vi "Compensazione.vi"(0 "Grandezza target":dbl, 1 "Grandezza reale letta":dbl, 2 "Precisione":dbl, 3 "Delta compensazione max":dbl, 4 "Time attesa stabilizzazione (s)":dbl, 5 "Grandezza attuale in":dbl, 6 "Reset comp?":bool, 7 "Compensazione abilitata":bool) -> (15 "compensazione":dbl, 17 "Grandezza stabilizz?":bool, 19 "Grandezza attuale out":dbl)   [LabVIEW 2019]
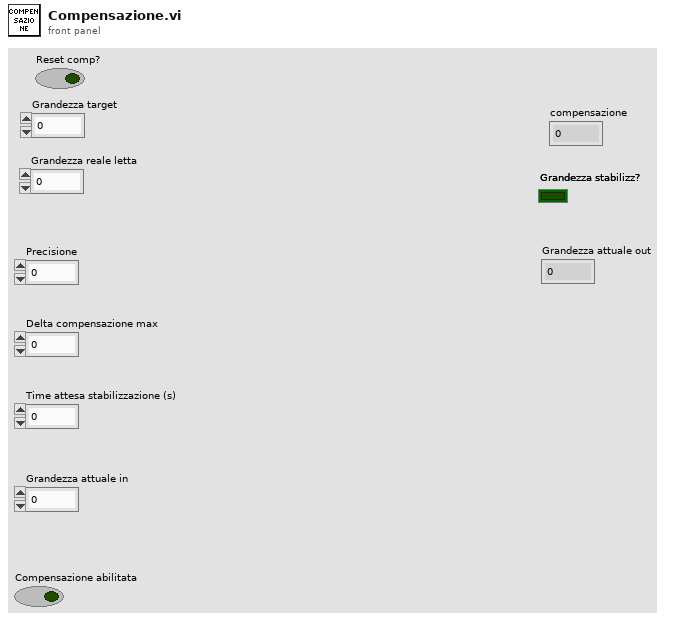
[diagram p1: front panel]
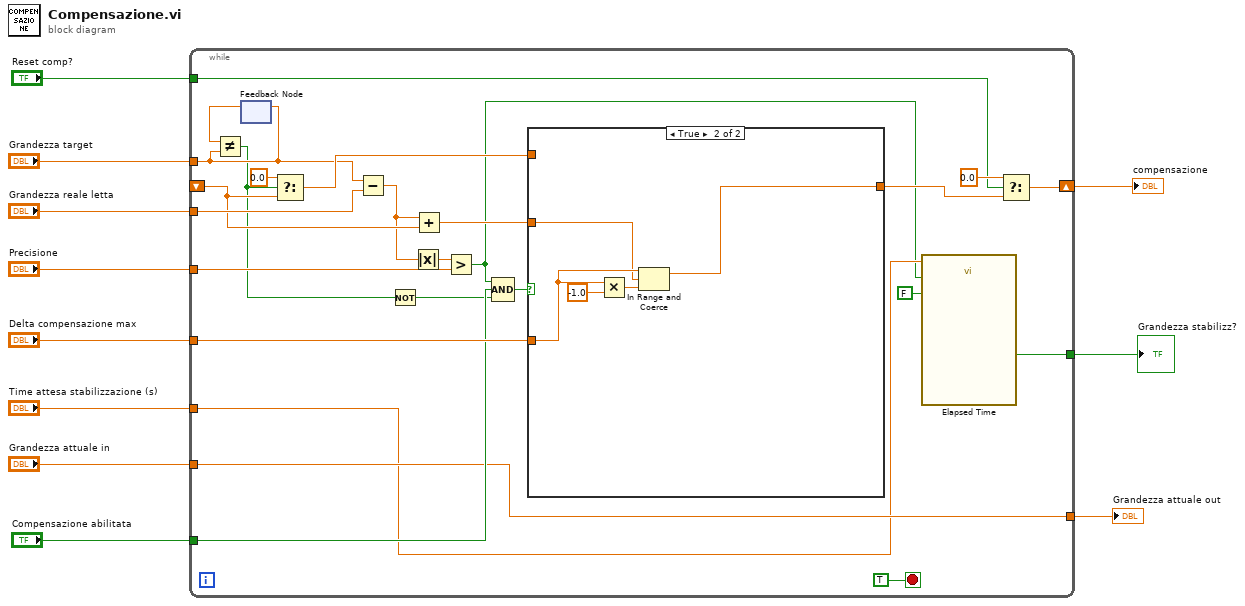
[diagram p0: block diagram]
diagram:
  n1 = while {
    tunnel: "Precisione" -> [w36]
    tunnel: "Grandezza attuale in" -> [w30]
    tunnel: "Compensazione abilitata" -> [w32]
    shift-right: [w21] -> w7
    shift-left: _ -> [w17]
    tunnel: "Delta compensazione max" -> [w34]
    tunnel: [w30] -> w6
    tunnel: "Grandezza target" -> [w18]
    tunnel: "Grandezza reale letta" -> [w29]
    tunnel: "Time attesa stabilizzazione (s)" -> [w27]
    tunnel: [w26] -> w2
    tunnel: "Reset comp?" -> [w19]
    stop <- TRUE stop-if-true
    n2 = feedback-in #1(w18) -> ()
    n3 = feedback #1() -> (w25:dbl)  [unwired: 1 in]
    n4 = Not Equal?(x=w25, y=w18) -> (x != y?=w14:bool)
    n5 = Select(t=0.0, s=w14, f=w17) -> (s? t:f=w24:dbl)
    n6 = Subtract(x=w18, y=w29) -> (x-y=w16:dbl)
    n7 = Not(x=w14) -> (.not. x?=w13:bool)
    n8 = Absolute Value(x=w16) -> (abs(x)=w33:dbl)
    n9 = Add(x=w16, y=w17) -> (x+y=w15:dbl)
    n10 = Greater?(x=w33, y=w36) -> (0:w12:bool)
    n11 = Compound Arithmetic op=AND(w12, w32, w13) -> (w31:bool)
    n12 = case shown="True" w31 {
      tunnel: w15 -> [_ w39]
      tunnel: [w37 w38] -> w22
      tunnel: w34 -> [_ w42]
      tunnel: w24 -> [w37 _]
      frame False {
      }
      frame True {
        n13 = Multiply(x=w42, y=-1.0) -> (x*y=w40:dbl)
        n14 = In Range and Coerce(upper limit=w42, x=w39, lower limit=w40) -> (coerced(x)=w38:dbl)  [unwired: 1 out]
      }
    }
    n15 = call "Elapsed Time"("Time Target (s)"=w27, "Reset"=w12, "Auto Reset"=FALSE) -> ("Time has Elapsed"=w26:bool)  [unwired: 9 in, 7 out]
    n16 = Select(t=0.0, s=w19, f=w22) -> (s? t:f=w21:dbl)
  }
  "Grandezza attuale out" <- w6
  "compensazione" <- w7
  "Grandezza stabilizz?" <- w2
